vi "perplexity.vi"(8 "error in (no error)":errorcluster, 11 "Interface_perplexity in":refnum<class "Interface_perplexity.lvclass">) -> (0 "error out":errorcluster, 2 "perplexity":dbl, 3 "Interface_perplexity out":refnum<class "Interface_perplexity.lvclass">)   [LabVIEW 2020, in "Interface_perplexity.lvclass"]
doc: "Calculate approximate perplexity for data X."
uses:
  Interface_perplexity.lvclass
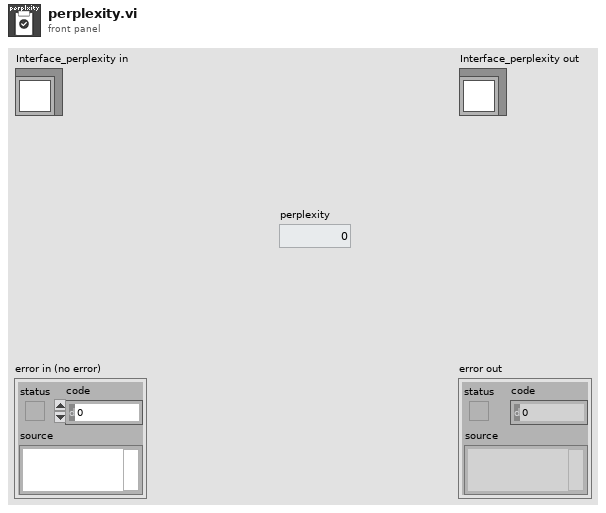
[diagram p1: front panel]
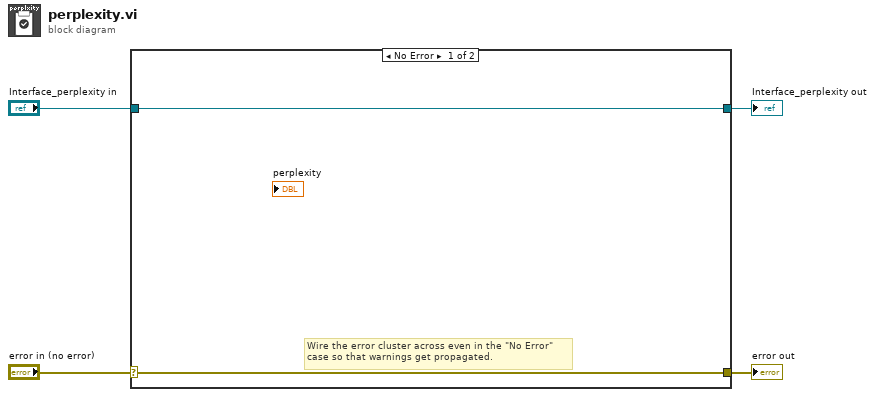
[diagram p0: block diagram]
diagram:
  n1 = case shown="No Error" "error in (no error)" {
    selector: "error in (no error)" -> [w5 w8]
    tunnel: [w5 w8] -> w3
    tunnel: [w6 w7] -> w1
    tunnel: "Interface_perplexity in" -> [w6 w7]
    frame No Error {
      # "Wire the error cluster across even in the \"No Error\"\ncase so that warnings get propagated."
    }
    frame Error {
    }
  }
  "error out" <- w3
  "Interface_perplexity out" <- w1
